vi "get done signal.vi"(8 "error in (no error)":errorcluster, 11 "Ixon_Ultra in":refnum<class "Ixon_Ultra.lvclass">) -> (0 "error out":errorcluster, 3 "Ixon_Ultra out":refnum<class "Ixon_Ultra.lvclass">)   [LabVIEW 2018, in "Ixon_Ultra.lvclass"]
uses:
  Ixon_Ultra.lvclass
  C:/Users/Denis/Desktop/S4ACS/S4ACS/Sim_Ixon_Ultra/Sim_Ixon_Ultra.lvclass
  Sim_Ixon_Ultra/Sim_Ixon_Ultra.lvclass/Sim_Ixon_Ultra.ctl
  Sim_Ixon_Ultra/Sim_Ixon_Ultra.lvclass
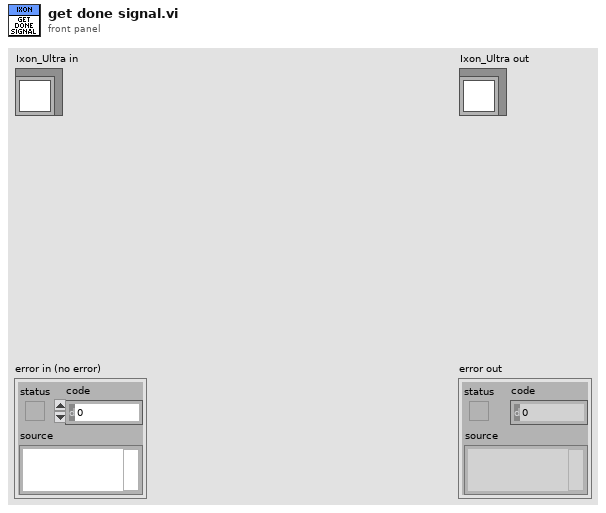
[diagram p1: front panel]
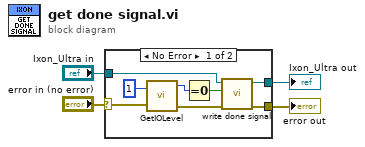
[diagram p0: block diagram]
diagram:
  n1 = case shown="No Error" "error in (no error)" {
    selector: "error in (no error)" -> [w12 w13]
    tunnel: "Ixon_Ultra in" -> [w10 w14]
    tunnel: [w9 w14] -> w2
    tunnel: [w8 w13] -> w1
    frame No Error {
      n2 = call <userlib>:"GetIOLevel.vi"("index"=1, "error in (no error)"=w12) -> ("iLevel"=w6:i32, "error out"=w7:errorcluster)  [unwired: 1 out]
      n3 = Equal To 0?(x=w6) -> (x = 0?=w5:bool)
      n4 = call "write done signal.vi"("error in (no error)"=w7, "done signal"=w5, "Sim_Ixon_Ultra in"=w10) -> ("error out"=w8:errorcluster, "Sim_Ixon_Ultra out"=w9:refnum<class "Ixon_Ultra.lvclass">)  [unwired: 7 in]
    }
    frame Error {
    }
  }
  "error out" <- w1
  "Ixon_Ultra out" <- w2
